vi "Sequence.CreateMainWhileLoop.vi"(8 "error in (no error)":errorcluster, 11 "Steps":T1[](array[typedef])) -> (0 "error out":errorcluster, 3 "WhileLoop Ref":refnum<k24>)   [LabVIEW 2015, in "Single Station Execution.lvlib"]
uses:
  Single Station Execution.lvlib
  Types/Compiled.StepProperties.ctl
  Types/Compiled.IOStateProperties.ctl
  Types/Compiled.StepElementProperties.ctl
  Types/Channel.Properties.ctl
  Types/Step.Types.ctl
  Types/Compiled.StepCondition.ctl
  Types/Conditions.OperationTypes.ctl
  NationalInstruments.VeriStand.RealTimeSequenceDefinitionApi
  Main.Constants.vi
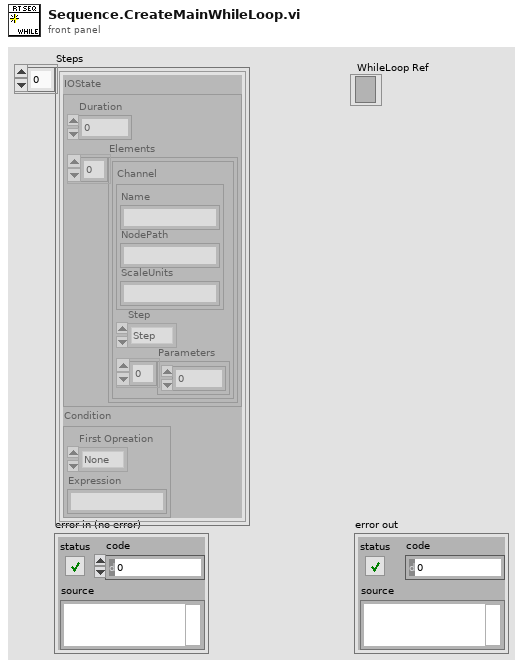
[diagram p1: front panel]
types:
  T1 = typedef "Single Station Execution.lvlib/Compiled.StepProperties.ctl" = cluster{"IOState":T2, "Condition":T6}
  T2 = typedef "Single Station Execution.lvlib/Compiled.IOStateProperties.ctl" = cluster{"Duration":dbl, "Elements":T3[]}
  T3 = typedef "Single Station Execution.lvlib/Compiled.StepElementProperties.ctl" = cluster{"Channel":T4, "Step":T5, "Parameters":dbl[]}
  T4 = typedef "Single Station Execution.lvlib/Channel.Properties.ctl" = cluster{"Name":string, "NodePath":string, "ScaleUnits":string}
  T5 = typedef "Single Station Execution.lvlib/Step.Types.ctl" = enum8{"Step", "iStep", "Ramp", "Unchanged", "Unknown", "Sine", "LogSine", "LinearSine", "ForcedRamp", "Waveform"}
  T6 = typedef "Single Station Execution.lvlib/Compiled.StepCondition.ctl" = cluster{"First Opreation":T7, "Expression":string}
  T7 = typedef "Single Station Execution.lvlib/Conditions.OperationTypes.ctl" = enum8{"None", "&&", "||"}
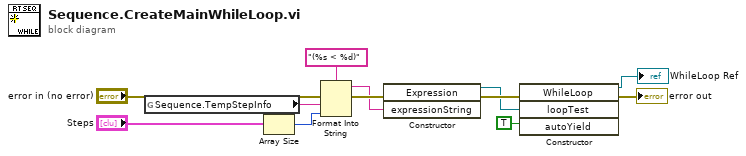
[diagram p0: block diagram]
diagram:
  n1 = global read "Main.Constants.vi" "Sequence.TempStepInfo"() -> (w12:string)
  n2 = Array Size(array="Steps") -> (size(s)=w11:i32)
  n3 = Format Into String(format string="(%s < %d)", error in="error in (no error)", w12, w11) -> (resulting string=w9:string, error out=w10:errorcluster)  [unwired: 1 in]
  n4 = constructor class="Expression"(error in=w10, "expressionString"=w9) -> (reference out=w3:refnum<k24>, error out=w7:errorcluster)  [unwired: 2 in, 2 out]
  n5 = constructor class="WhileLoop"(error in=w7, "loopTest"=w3, "autoYield"=TRUE) -> (reference out=→"WhileLoop Ref":refnum<k24>, error out=→"error out":errorcluster)  [unwired: 2 in, 3 out]
